vi "Write Depth Scale.vi"(8 "error in (no error)":errorcluster, 10 "Depth Scale":dbl, 11 "Video File in":refnum<class "Video File.lvclass">) -> (0 "error out":errorcluster, 3 "Video File out":refnum<class "Video File.lvclass">)   [LabVIEW 2018, in "Video File.lvclass"]
uses:
  Video File.lvclass
  Video File.lvclass/Video File.ctl
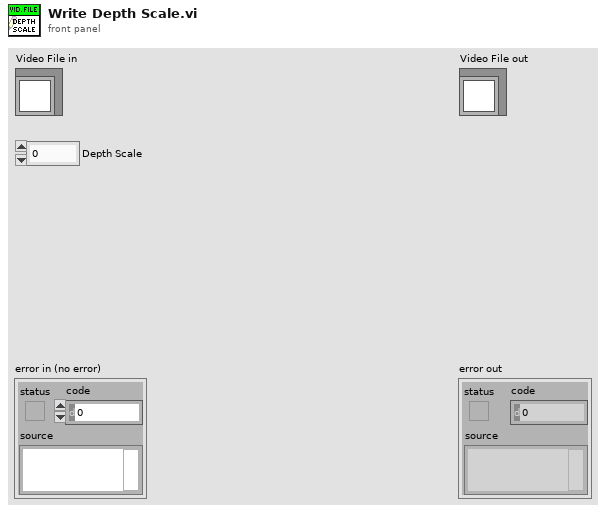
[diagram p1: front panel]
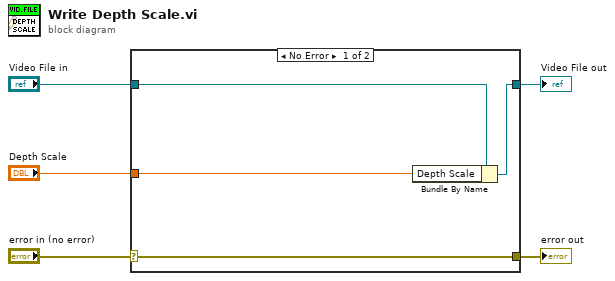
[diagram p0: block diagram]
diagram:
  n1 = case shown="No Error" "error in (no error)" {
    selector: "error in (no error)" -> [w9 w10]
    tunnel: [w9 w10] -> w4
    tunnel: [w7 w11] -> w2
    tunnel: "Video File in" -> [w8 w11]
    tunnel: "Depth Scale" -> [w6 _]
    frame No Error {
      n2 = Bundle By Name(cluster=w8, "Depth Scale"=w6) -> (w7:refnum<class "Video File.lvclass">)
    }
    frame Error {
    }
  }
  "error out" <- w4
  "Video File out" <- w2
